vi "ControlFunction.vi"(8 "error in (no error)":errorcluster, 11 "Intake in":refnum<class "Intake.lvclass">) -> (0 "error out":errorcluster, 3 "Intake out":refnum<class "Intake.lvclass">)   [LabVIEW 2017, in "Intake.lvclass"]
uses:
  Intake.lvclass
  SubsystemData/IntakeData/IntakeData.lvclass
  R:/Documents/github/FRC4080/2018-robot-main/SubsystemData/SubsystemData.lvclass
  Team-code/IntakeOutput.ctl
  <vilib>/Rock Robotics/WPI/ThirdParty/Phoenix-LabVIEW/Motor Controller/Controls/CTRE_Phoenix_MotorControl_ControlMode.ctl
  Intake.lvclass/Intake.ctl
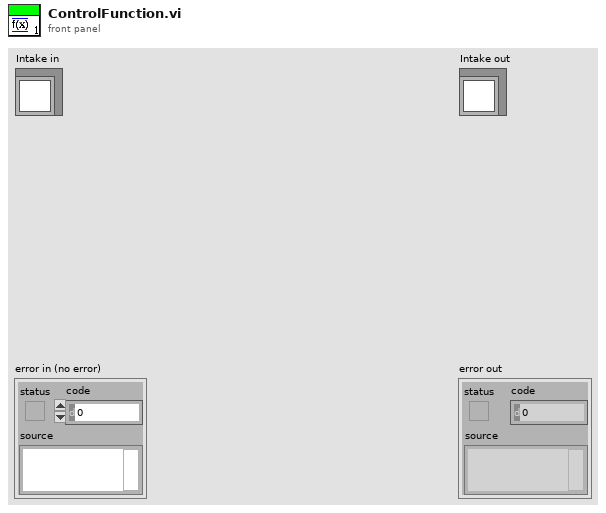
[diagram p1: front panel]
types:
  T1 = typedef "IntakeData.lvclass/IntakeOutput.ctl" = cluster{"Control Mode":T2, "LeftIntakeSetting":dbl, "RightIntakeSetting":dbl}
  T2 = typedef "CTRE_Phoenix_MotorControl_ControlMode.ctl" = u16
  T3 = typedef "IntakeData.lvclass/IntakeCommand.ctl" = cluster{"Collect":bool, "Deposit":bool}
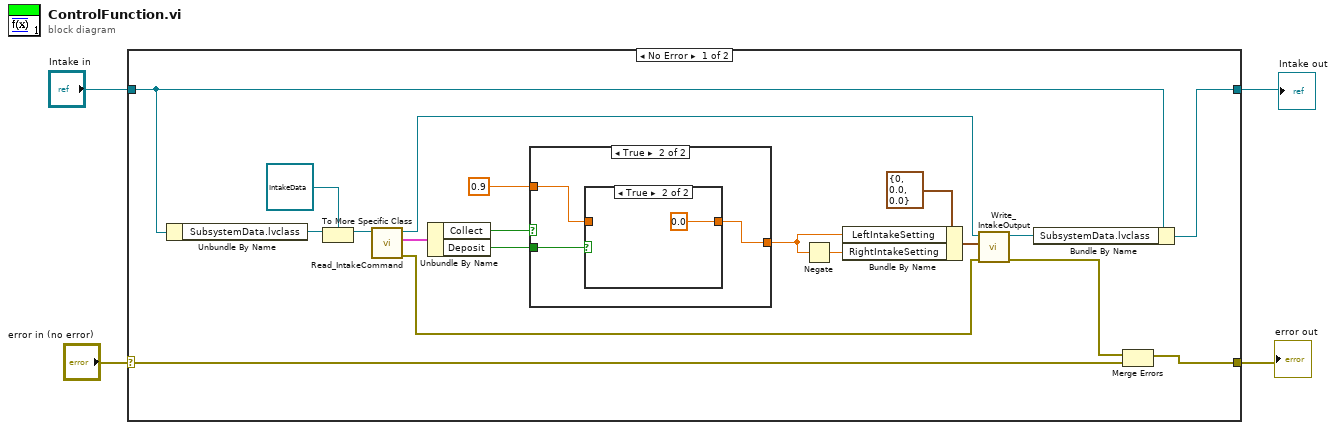
[diagram p0: block diagram]
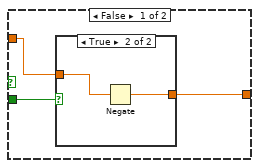
[diagram p2: hidden frame]
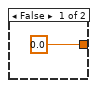
[diagram p3: hidden frame]
diagram:
  n1 = case shown="No Error" "error in (no error)" {
    selector: "error in (no error)" -> [w23 w36]
    tunnel: [w20 w36] -> w3
    tunnel: [w22 w35] -> w1
    tunnel: "Intake in" -> [w21 w35]
    frame No Error {
      n2 = Unbundle By Name(w21) -> ("SubsystemData.lvclass"=w18:refnum<class "SubsystemData.lvclass">)
      n3 = To More Specific Class(target class=refnum<class "IntakeData.lvclass"> refnum ("IntakeData.lvclass"), reference=w18) -> (specific class reference=w17:refnum<class "IntakeData.lvclass">)  [unwired: 1 in, 1 out]
      n4 = call-dynamic "Read_IntakeCommand.vi"("IntakeData in"=w17) -> ("error out"=w14:errorcluster, "Intake Command"=w12:T3, "IntakeData out"=w15:refnum<class "IntakeData.lvclass">)  [unwired: 8 in]
      n5 = Unbundle By Name(w12) -> ("Collect"=w8:bool, "Deposit"=w7:bool)
      n6 = case shown="True" w8 {
        tunnel: w7 -> [w26 w32]
        tunnel: [w24 w31] -> w6
        tunnel: 0.9 -> [w25 w30]
        frame False {
          n7 = case shown="True" w26 {
            tunnel: w25 -> [_ w29]
            tunnel: [0.0 w28] -> w24
            frame False {
            }
            frame True {
              n8 = Negate(x=w29) -> (-x=w28:dbl)
            }
          }
        }
        frame True {
          n9 = case shown="True" w32 {
            tunnel: [w33 0.0] -> w31
            tunnel: w30 -> [w33 _]
            frame False {
            }
            frame True {
            }
          }
        }
      }
      n10 = Negate(x=w6) -> (-x=w9:dbl)
      n11 = Bundle By Name(cluster=T1 {"Control Mode"=0, "LeftIntakeSetting"=0.0, "RightIntakeSetting"=0.0} ("IntakeOutput"), "LeftIntakeSetting"=w6, "RightIntakeSetting"=w9) -> (w11:T1)
      n12 = call-dynamic "Write_IntakeOutput.vi"("error in (no error)"=w14, "IntakeOutput"=w11, "IntakeData in"=w15) -> ("error out"=w13:errorcluster, "IntakeData out"=w19:refnum<class "IntakeData.lvclass">)  [unwired: 7 in]
      n13 = Bundle By Name(cluster=w21, "SubsystemData.lvclass"=w19) -> (w22:refnum<class "Intake.lvclass">)
      n14 = Merge Errors(w13, w23) -> (w20:errorcluster)
    }
    frame Error {
    }
  }
  "error out" <- w3
  "Intake out" <- w1
